vi "Get and Set FP Width and Height.vi"(7 "Select":enum16{"WinBounds", "PanelBounds"}(ring)=enum."PanelBounds", 8 "错误输入（无错误）":errorcluster, 9 "Mode":enum16{"Read", "Write"}(ring), 10 "Bounds In":cluster{"Width":i16, "Height":i16}, 11 "VI Ref In":refnum<vi>) -> (0 "错误输出":errorcluster, 2 "Bounds Out":cluster{"Left":i16, "Right":i16}, 3 "VI Ref Out":refnum<vi>)   [LabVIEW 2012, in "VIRef.lvlib"]
uses:
  VIRef.lvlib
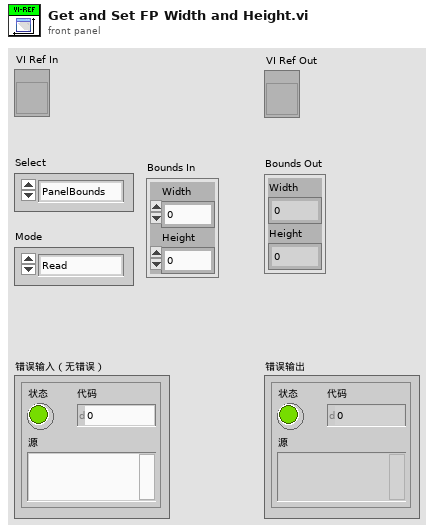
[diagram p1: front panel]
types:
  T1 = typedef "LVRectTypeDef.ctl" = cluster{"Left":i16, "Top":i16, "Right":i16, "Bottom":i16}
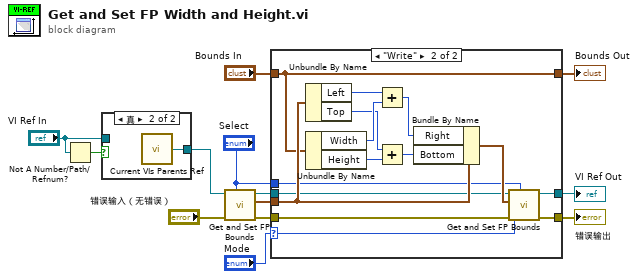
[diagram p0: block diagram]
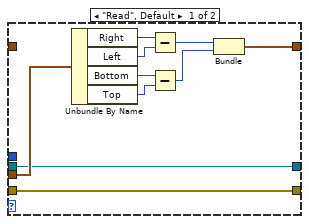
[diagram p2: hidden frame]
diagram:
  n1 = Not A Number/Path/Refnum?(number/path/refnum="VI Ref In") -> (NaN/Path/Refnum?=w13:bool)
  n2 = case shown="真" w13 {
    tunnel: [w14 w15] -> w10
    tunnel: "VI Ref In" -> [w14 _]
    frame False {
    }
    frame True {
      n3 = call "Current VIs Parents Ref.vi"() -> ("Calling VI's Reference"=w15:refnum<vi>)  [unwired: 2 in]
    }
  }
  n4 = call "Get and Set FP Bounds.vi"("Select"="Select", "错误输入（无错误）"="错误输入（无错误）", "VI Ref In"=w10) -> ("错误输出"=w8:errorcluster, "Bounds Out"=w6:T1, "VI Ref Out"=w2:refnum<vi>)  [unwired: 6 in]
  n5 = case shown="\"Write\"" "Mode" {
    selector: "Mode" -> [_ w30]
    tunnel: w8 -> [w25 w29]
    tunnel: [w25 w28] -> w7
    tunnel: w6 -> [w18 w40]
    tunnel: "Bounds In" -> [_ w33]
    tunnel: [w17 w33] -> w4
    tunnel: "Select" -> [_ w31]
    tunnel: w2 -> [w16 w27]
    tunnel: [w16 w26] -> w1
    frame "Read", Default {
      n6 = Unbundle By Name(w18) -> ("Right"=w20:i16, "Left"=w19:i16, "Bottom"=w21:i16, "Top"=w22:i16)
      n7 = Subtract(x=w20, y=w19) -> (x-y=w23:i16)
      n8 = Subtract(x=w21, y=w22) -> (x-y=w24:i16)
      n9 = Bundle(w23, w24) -> (w17:cluster{i16, i16})  [unwired: 1 in]
    }
    frame "Write" {
      n10 = Unbundle By Name(w40) -> ("Left"=w39:i16, "Top"=w36:i16)
      n11 = Unbundle By Name(w33) -> ("Width"=w38:i16, "Height"=w35:i16)
      n12 = Add(x=w39, y=w38) -> (x+y=w37:i16)
      n13 = Add(x=w36, y=w35) -> (x+y=w34:i16)
      n14 = Bundle By Name(cluster=w40, "Right"=w37, "Bottom"=w34) -> (w32:T1)
      n15 = call "Get and Set FP Bounds.vi"("Select"=w31, "错误输入（无错误）"=w29, "Mode"=w30, "Bounds In"=w32, "VI Ref In"=w27) -> ("错误输出"=w28:errorcluster, "VI Ref Out"=w26:refnum<vi>)  [unwired: 4 in, 1 out]
    }
  }
  "VI Ref Out" <- w1
  "错误输出" <- w7
  "Bounds Out" <- w4
